vi "TestExampleAB.vi"   [LabVIEW 2012]
doc: "Test VI demonstrating the interplay of the example classes."
uses:
  ExampleClassA/ExampleClassA.lvclass
  ExampleClassB/ExampleClassB.lvclass
  <vilib>/Distrio/Murmex/Murmex/Murmex.lvclass
panel:
  # "Test Example A & B"
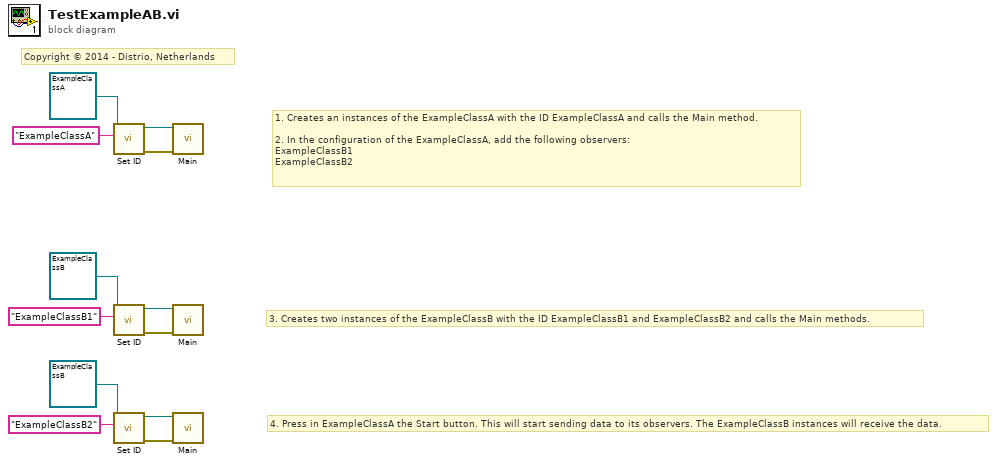
[diagram p0: block diagram]
diagram:
  # "4. Press in ExampleClassA the Start button. This will start sending data to its observers. The ExampleClassB instances will receive the data."
  # "3. Creates two instances of the ExampleClassB with the ID ExampleClassB1 and ExampleClassB2 and calls the Main methods."
  # "1. Creates an instances of the ExampleClassA with the ID ExampleClassA and calls the Main method.\n\n2. In the configuration of the ExampleClassA, add the following observers:\nExampleClassB1\nExampleClassB2"
  # "Copyright © 2014 - Distrio, Netherlands"
  n1 = call <vilib>:"Set ID.vi"("id"="ExampleClassA", "Murmex in"=refnum<class "ExampleClassA.lvclass"> refnum ("ExampleClassA.lvclass")) -> ("error out"=w10:errorcluster, "Murmex out"=w9:refnum<class "ExampleClassA.lvclass">)  [unwired: 8 in]
  n2 = call <vilib>:"Set ID.vi"("id"="ExampleClassB1", "Murmex in"=refnum<class "ExampleClassB.lvclass"> refnum ("ExampleClassB.lvclass")) -> ("error out"=w5:errorcluster, "Murmex out"=w6:refnum<class "ExampleClassB.lvclass">)  [unwired: 8 in]
  n3 = call <vilib>:"Set ID.vi"("id"="ExampleClassB2", "Murmex in"=refnum<class "ExampleClassB.lvclass"> refnum ("ExampleClassB.lvclass")) -> ("error out"=w4:errorcluster, "Murmex out"=w3:refnum<class "ExampleClassB.lvclass">)  [unwired: 8 in]
  n4 = call-dynamic "Main.vi"("error in (no error)"=w10, "Example Class A in"=w9) -> ()  [unwired: 8 in, 2 out]
  n5 = call-dynamic "Main.vi"("error in (no error)"=w5, "Example Class B in"=w6) -> ()  [unwired: 8 in, 2 out]
  n6 = call-dynamic "Main.vi"("error in (no error)"=w4, "Example Class B in"=w3) -> ()  [unwired: 8 in, 2 out]
